vi "Initialisation COM RS.vi"(6 "Enable Termination\nChar (T)":bool, 7 "termination char\n(0xA = '\\n' = LF)":u8=10 caption="car. de terminaison\n(0xA = 'n' = LF)" format="%.0x", 8 "entrée d'erreur (pas d'erreur)":errorcluster, 10 "baud rate (9600)":i32=9600, 11 "Refnum VISA en entrée":refnum<visa-resource-name>) -> (0 "sortie d'erreur":errorcluster, 3 "Nom de ressource VISA en sortie":refnum<visa-resource-name>)   [LabVIEW 2020]
uses:
  <vilib>/Instr/_visa.llb/VISA Set IO Buffer Mask.ctl
  <vilib>/Instr/_visa.llb/VISA Configure Serial Port (Instr).vi
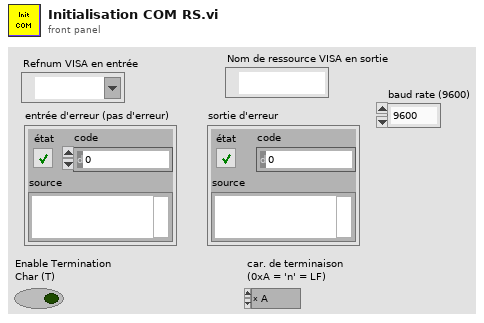
[diagram p1: front panel]
types:
  T1 = typedef "VISA Set IO Buffer Mask.ctl" = u16
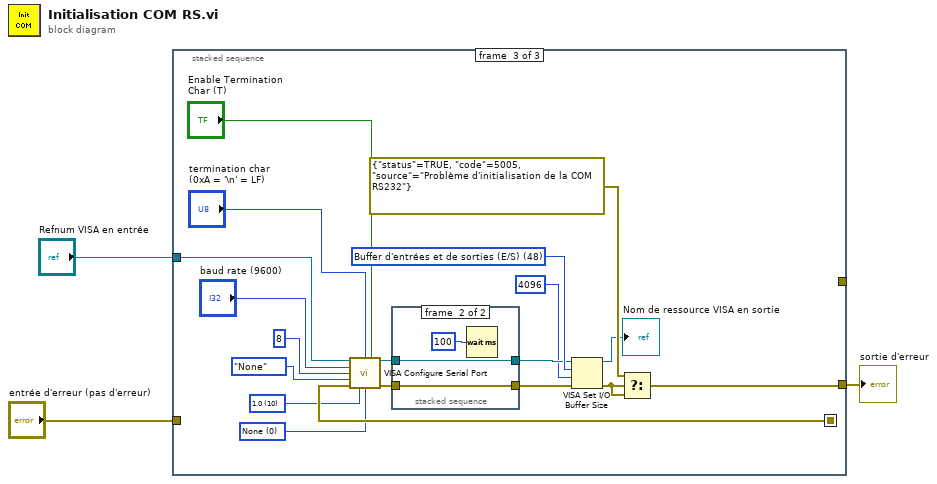
[diagram p0: block diagram]
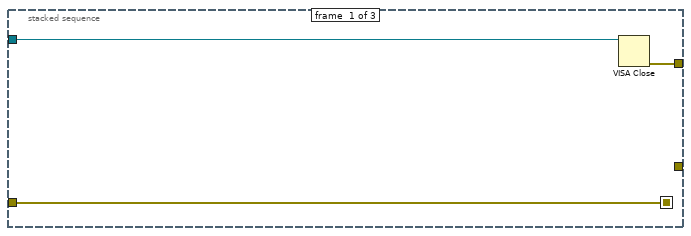
[diagram p2: hidden frame]
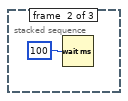
[diagram p3: hidden frame]
diagram:
  n1 = stacked-sequence {
    seq-local: [w6 _ _] -> [_ _ w25]
    tunnel: "entrée d'erreur (pas d'erreur)" -> [w6 _ _]
    tunnel: [_ _ w26] -> w3
    tunnel: "Refnum VISA en entrée" -> [w5 _ w9]
    tunnel: [w4 _ _] -> _
    frame #0 {
      n2 = VISA Close(VISA resource name=w5) -> (error out=w4:errorcluster)  [unwired: 1 in]
    }
    frame #1 {
      n3 = Wait (ms)(milliseconds to wait=u32 100 ("attente (ms)")) -> ()  [unwired: 1 out]
    }
    frame #2 {
      w22 = T1 48 items=["Buffer d'entrées (E/S)"=16, "Buffer de sorties (E/S)"=32, "Buffer d'entrées et de sorties (E/S)"=48] ("Mask")
      w11 = u16 0 items=["None", "XON/XOFF", "RTS/CTS", "XON/XOFF & RTS/CTS", "DTR/DSR", "XON/XOFF & DTR/DSR"] ("flow control (0:none)")
      w12 = u16 10 items=["1.0"=10, "1.5"=15, "2.0"=20] ("stop bits (10: 1 bit)")
      n4 = call-poly "VISA Configure Serial Port"("VISA resource name"=w9, "termination char\n(0xA = '\\n' = LF)"="termination char\n(0xA = '\\n' = LF)", "Enable Termination\nChar (T)"="Enable Termination\nChar (T)", "baud rate (9600)"="baud rate (9600)", "data bits (8)"=u16 8, "parity (0:none)"=enum16{"None", "Odd", "Even", "Mark", "Space"}."None", "error in (no error)"=w25, "stop bits (10: 1 bit)"=w12, "flow control (0:none)"=w11) -> ("VISA resource name out"=w17:refnum<visa-resource-name>, "error out"=w20:errorcluster)  [unwired: 5 in]
      n5 = stacked-sequence {
        tunnel: w17 -> [_ w29]
        tunnel: [_ w29] -> w18
        tunnel: [_ w28] -> w19
        tunnel: w20 -> [_ w28]
        frame #0 {
        }
        frame #1 {
          n6 = Wait (ms)(milliseconds to wait=u32 100) -> ()  [unwired: 1 out]
        }
      }
      n7 = VISA Set I/O Buffer Size(VISA resource name=w18, mask (16)=w22, size (4096)=u32 4096 ("taille (4096)"), error in (no error)=w19) -> (VISA resource name out=→"Nom de ressource VISA en sortie":refnum<visa-resource-name>, error out=w15:errorcluster)
      n8 = Select(t=errorcluster {"status"=TRUE, "code"=5005, "source"="Problème d'initialisation de la COM RS232"} ("cas vrai"), s=w15, f=w15) -> (s? t:f=w26:errorcluster)
    }
  }
  "sortie d'erreur" <- w3
